vi "Query Builder - Dynamic Columns.vi"(8 "Date-Time Column Name":string="Date-Time", 11 "Query Build Cluster":T1={"Sample Check box"=TRUE, "Sample Comparison Type"="Is exactly", "Sample Name"="", "Logical Sample-Lot "="OR", "LotID Checkbox"=TRUE, "Lot Comparison Type"="Is exactly", "LotID Name"="", "Logical Lot-Date"="OR", "Date Checkbox"=TRUE, "Start Date"=timestamp(3375812149.928578 s since 1904-01-01), "End Date"=timestamp(3375812149.928578 s since 1904-01-01), "1st search column name"="", "2nd search column name"=""} {"Start Date" format="%<%X\n%x>T"; "End Date" format="%<%X\n%x>T"}) -> (3 "Where Statement":string=" WHERE (  CryoProber_MCT_Std_Sample_Summary.Sample_Name  = '' OR  Lot_ID  = '' OR [Date-Time] BETWEEN CONVERT (Datetime, '12/21/2010 15:35:49') AND CONVERT (Datetime, '12/21/2010 15:35:49') ) ")   [LabVIEW 2010]
panel:
  # "Get all results where"
  # "where"
  # "between these dates"
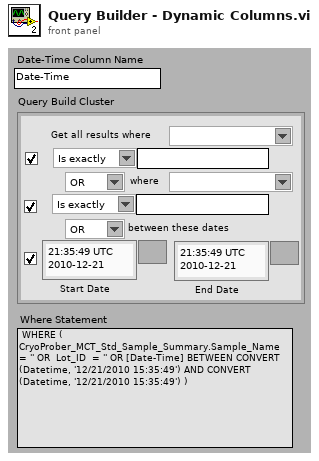
[diagram p1: front panel]
types:
  T1 = cluster{"Sample Check box":bool, "Sample Comparison Type":string, "Sample Name":string, "Logical Sample-Lot ":string, "LotID Checkbox":bool, "Lot Comparison Type":string, "LotID Name":string, "Logical Lot-Date":string, "Date Checkbox":bool, "Start Date":timestamp, "End Date":timestamp, "1st search column name":string, "2nd search column name":string}
  T2 = enum16{"MS SQL Format", "Access Format", "Using CONVERT func", "Using # # "}
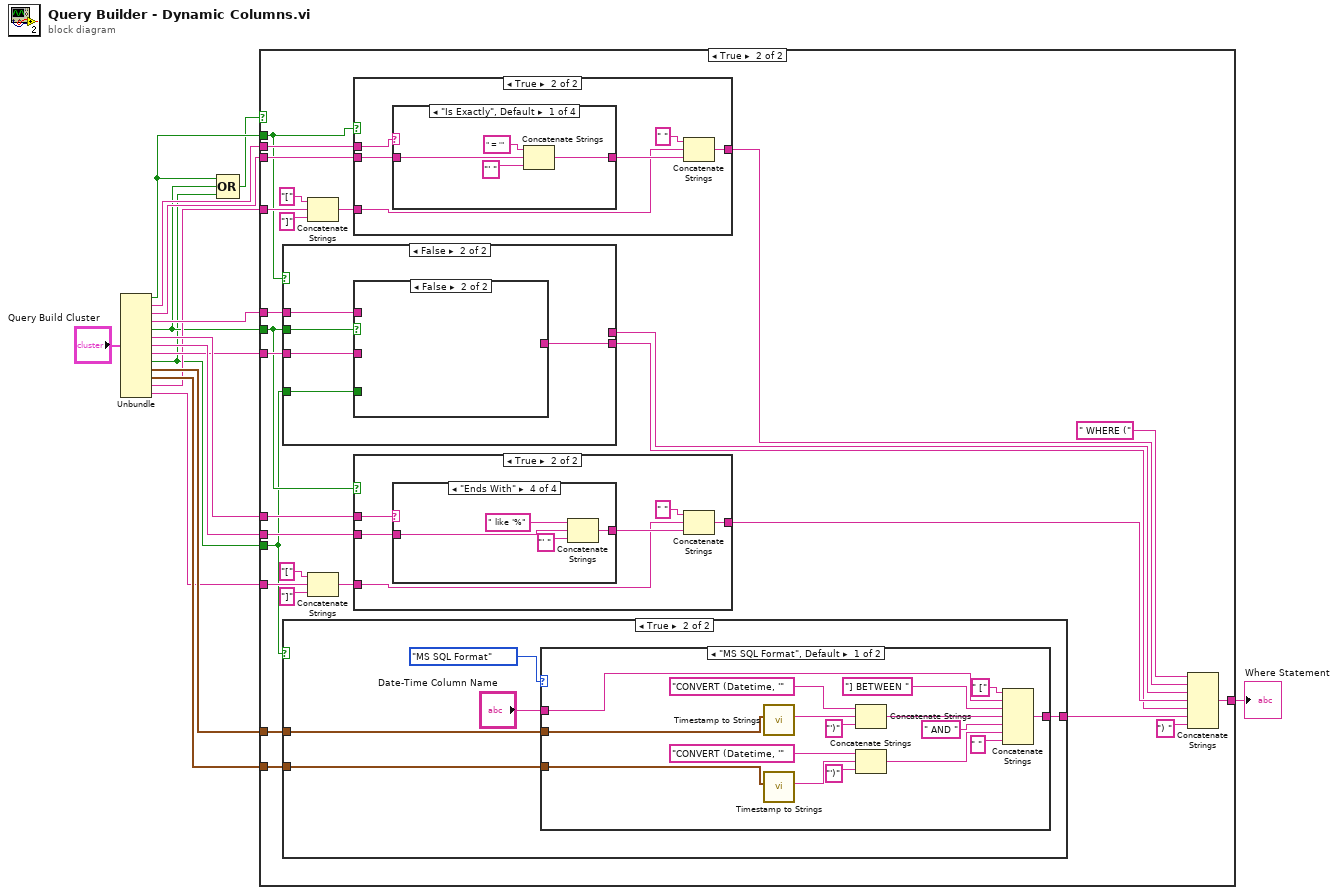
[diagram p0: block diagram]
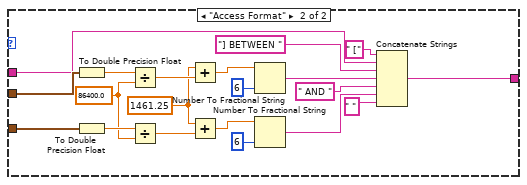
[diagram p4: hidden frame]
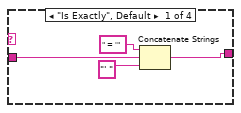
[diagram p6: hidden frame]
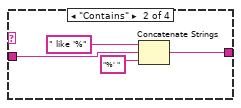
[diagram p7: hidden frame]
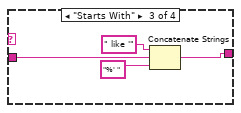
[diagram p8: hidden frame]
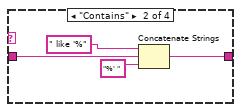
[diagram p10: hidden frame]
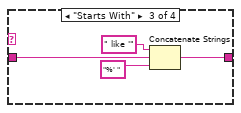
[diagram p11: hidden frame]
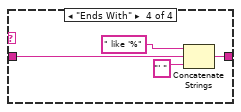
[diagram p12: hidden frame]
diagram:
  n1 = Unbundle("Query Build Cluster") -> ("Sample Check box"=w4:bool, "Sample Comparison Type"=w15:string, "Sample Name"=w14:string, "Logical Sample-Lot"=w13:string, "LotID Checkbox"=w3:bool, "Lot Comparison Type"=w12:string, "LotID Name"=w11:string, "Logical Lot-Date"=w10:string, "Date Checkbox"=w2:bool, "Start Date"=w9:timestamp, "End Date"=w8:timestamp, "1st search column name"=w6:string, "2nd search column name"=w5:string)
  n2 = Compound Arithmetic op=OR(w4, w3, w2) -> (w1:bool)
  n3 = case shown="True" w1 {
    tunnel: w15 -> [_ w37]
    tunnel: w14 -> [_ w36]
    tunnel: w13 -> [_ w35]
    tunnel: w12 -> [_ w34]
    tunnel: w11 -> [_ w33]
    tunnel: w10 -> [_ w32]
    tunnel: w9 -> [_ w31]
    tunnel: w8 -> [_ w30]
    tunnel: [_ w29] -> w7
    tunnel: w6 -> [_ w25]
    tunnel: w5 -> [_ w22]
    tunnel: w4 -> [_ w19]
    tunnel: w3 -> [_ w18]
    tunnel: w2 -> [_ w17]
    frame False {
    }
    frame True {
      n4 = case shown="False" w19 {
        tunnel: w18 -> [w134 w149]
        tunnel: w17 -> [w133 w148]
        tunnel: w35 -> [w132 w147]
        tunnel: [w131 _] -> w41
        tunnel: w32 -> [w130 w146]
        tunnel: [w129 w145] -> w39
        frame True {
          n5 = case shown="False" w134 {
            tunnel: w133 -> [w138 w143]
            tunnel: w132 -> [w137 w141]
            tunnel: [w137 w140] -> w131
            tunnel: w130 -> [w136 w142]
            tunnel: [w135 _] -> w129
            frame True {
              n6 = case shown="True" w138 {
                tunnel: w136 -> [_ w139]
                tunnel: [_ w139] -> w135
                frame False {
                }
                frame True {
                }
              }
            }
            frame False {
              n7 = case shown="True" w143 {
                tunnel: w142 -> [_ _]
                tunnel: w141 -> [_ w144]
                tunnel: [_ w144] -> w140
                frame False {
                }
                frame True {
                }
              }
            }
          }
        }
        frame False {
          n8 = case shown="False" w149 {
            tunnel: w148 -> [w152 _]
            tunnel: w147 -> [_ _]
            tunnel: w146 -> [w151 _]
            tunnel: [w150 _] -> w145
            frame True {
              n9 = case shown="False" w152 {
                tunnel: w151 -> [_ w153]
                tunnel: [_ w153] -> w150
                frame False {
                }
                frame True {
                }
              }
            }
            frame False {
            }
          }
        }
      }
      n10 = case shown="True" w17 {
        tunnel: [_ w48] -> w38
        tunnel: w31 -> [_ w46]
        tunnel: w30 -> [_ w47]
        frame False {
        }
        frame True {
          n11 = case shown="\"MS SQL Format\", Default" T2."MS SQL Format" {
            tunnel: [w61 w81] -> w48
            tunnel: w47 -> [w50 w79]
            tunnel: w46 -> [w54 w77]
            tunnel: "Date-Time Column Name" -> [w59 w65]
            frame "MS SQL Format", Default {
              n12 = call "Timestamp to Strings.vi"("Input Time"=w54) -> ("DB Date-Time"=w55:string)  [unwired: 3 in, 3 out]
              n13 = call "Timestamp to Strings.vi"("Input Time"=w50) -> ("DB Date-Time"=w49:string)  [unwired: 3 in, 3 out]
              n14 = Concatenate Strings("CONVERT (Datetime, '" ("string"), w55, "')" ("string")) -> (w56:string)
              n15 = Concatenate Strings("CONVERT (Datetime, '" ("string"), w49, "')" ("string")) -> (w51:string)
              n16 = Concatenate Strings(" [" ("string"), w59, "] BETWEEN " ("string"), w56, " AND " ("string"), w51, " " ("string")) -> (w61:string)
            }
            frame "Access Format" {
              w67 = 1461.25 ("x")
              w66 = 86400.0 ("y")
              n17 = To Double Precision Float(number=w77) -> (double precision float=w75:dbl)
              n18 = To Double Precision Float(number=w79) -> (double precision float=w74:dbl)
              n19 = Divide(x=w75, y=w66) -> (x/y=w78:dbl)
              n20 = Divide(x=w74, y=w66) -> (x/y=w76:dbl)
              n21 = Add(x=w67, y=w78) -> (x+y=w71:dbl)
              n22 = Add(x=w67, y=w76) -> (x+y=w70:dbl)
              n23 = Number To Fractional String(number=w71, precision (6)=i16 6) -> (F-format string=w69:string)  [unwired: 2 in]
              n24 = Number To Fractional String(number=w70, precision (6)=i16 6) -> (F-format string=w68:string)  [unwired: 2 in]
              n25 = Concatenate Strings(" [" ("string"), w65, "] BETWEEN " ("string"), w69, " AND " ("string"), w68, " " ("string")) -> (w81:string)
            }
          }
        }
      }
      n26 = Concatenate Strings("[" ("string"), w25, "]" ("string")) -> (w21:string)
      n27 = Concatenate Strings("[" ("string"), w22, "]" ("string")) -> (w20:string)
      n28 = case shown="True" w19 {
        tunnel: [_ w111] -> w42
        tunnel: w36 -> [_ w110]
        tunnel: w37 -> [_ w109]
        tunnel: w21 -> [_ w107]
        frame False {
        }
        frame True {
          n29 = case shown="\"Is Exactly\", Default" w109 {
            tunnel: [w114 w118 w122 w126] -> w112
            tunnel: w110 -> [w113 w117 w121 w125]
            frame "Is Exactly", Default {
              n30 = Concatenate Strings(" = '" ("string"), w113, "' " ("string")) -> (w114:string)
            }
            frame "Contains" {
              n31 = Concatenate Strings(" like '%" ("string"), w117, "%' " ("string")) -> (w118:string)
            }
            frame "Starts With" {
              n32 = Concatenate Strings(" like '" ("string"), w121, "%' " ("string")) -> (w122:string)
            }
            frame "Ends With" {
              n33 = Concatenate Strings(" like '%" ("string"), w125, "' " ("string")) -> (w126:string)
            }
          }
          n34 = Concatenate Strings(" " ("string"), w107, w112) -> (w111:string)
        }
      }
      n35 = case shown="True" w18 {
        tunnel: w34 -> [_ w90]
        tunnel: w33 -> [_ w89]
        tunnel: [_ w87] -> w40
        tunnel: w20 -> [_ w85]
        frame False {
        }
        frame True {
          n36 = case shown="\"Ends With\"" w90 {
            tunnel: [w92 w96 w100 w104] -> w88
            tunnel: w89 -> [w91 w95 w99 w103]
            frame "Is Exactly", Default {
              n37 = Concatenate Strings(" = '" ("string"), w91, "' " ("string")) -> (w92:string)
            }
            frame "Contains" {
              n38 = Concatenate Strings(" like '%" ("string"), w95, "%' " ("string")) -> (w96:string)
            }
            frame "Starts With" {
              n39 = Concatenate Strings(" like '" ("string"), w99, "%' " ("string")) -> (w100:string)
            }
            frame "Ends With" {
              n40 = Concatenate Strings(" like '%" ("string"), w103, "' " ("string")) -> (w104:string)
            }
          }
          n41 = Concatenate Strings(" " ("string"), w85, w88) -> (w87:string)
        }
      }
      n42 = Concatenate Strings(" WHERE (" ("string"), w42, w41, w40, w39, w38, ") " ("string")) -> (w29:string)
    }
  }
  "Where Statement" <- w7
